vi "steuerprogramm-2.vi"() -> ()   [LabVIEW 2010]
uses:
  GVtdms.vi
  GVAbschalten.vi
  <vilib>/rvi/interface/nirviReadWriteControl/nirviReadWriteControl.xnode
  C:/Users/HAGAR-IV/Desktop/Zeugs/Johnny/pertrasgc fpga/fpga-programm-2.vi
  <vilib>/rvi/interface/nirviCloseFPGA/nirviCloseFPGA.xnode
  <vilib>/RVI Host/nirviSupport.llb/nirviErrorClusterFromErrorCode.vi
  <vilib>/rvi/errors/niLvFpgaWhatHappensToTopLevelVI.ctl
  <vilib>/rvi/interface/common/niFpgaNodeNameForErrorReporting.ctl
  <vilib>/rvi/errors/niLvFpgaAdjustHostInterfaceError.vi
  <vilib>/FPGAPlugInAG/cRIO-9114/niLvFpga_Close_cRIO-9114.vi
panel:
  in  "Pfad":path
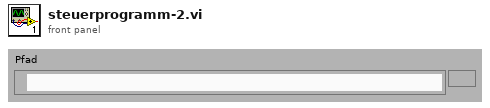
[diagram p1: front panel]
types:
  T1 = enum16{"open", "open or create", "create or replace", "create", "open (read-only)"}
  T2 = typedef "niFpgaNodeNameForErrorReporting.ctl" = enum16{"Open FPGA VI Reference", "Read/Write Control", "Invoke Method: Abort", "Invoke Method: Acknowledge IRQ", "Invoke Method: Download", "Invoke Method: FIFO.Configure", "Invoke Method: FIFO.Read", "Invoke Method: FIFO.Start", "Invoke Method: FIFO.Stop", "Invoke Method: FIFO.Write", "Invoke Method: Reset", "Invoke Method: Run", "Invoke Method: Wait on IRQ", "Close FPGA VI Reference"}
  T3 = typedef "niLvFpgaWhatHappensToTopLevelVI.ctl" = enum16{"top level VI scripted behind XNode", "top level VI inlined behind XNode"}
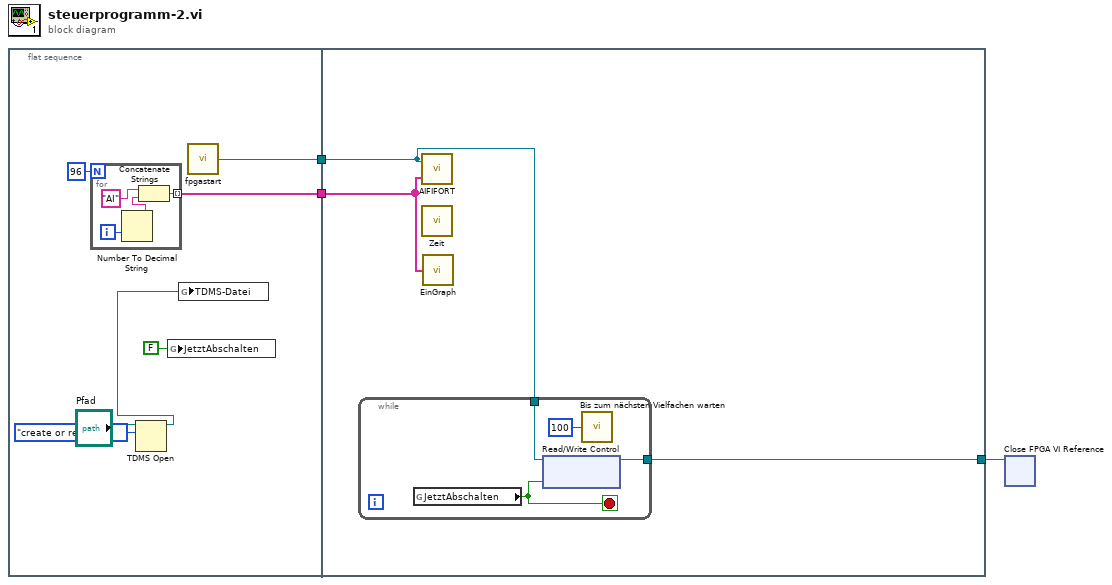
[diagram p0: block diagram]
diagram:
  n1 = flat-sequence {
    tunnel: [w10] -> w3
    tunnel: [w7] -> w1
    tunnel: w3 -> [w17]
    tunnel: [w16] -> w2
    tunnel: w1 -> [w15]
    frame #0 {
      n2 = for {
        N: 96 -> [_]
        tunnel: [w11] -> w7 mode=indexing
        i -> [w14]
        n3 = Number To Decimal String(number=w14) -> (decimal integer string=w12:string)  [unwired: 1 in]
        n4 = Concatenate Strings("AI", w12) -> (w11:string)
      }
      n5 = TDMS Open(10:T1."create or replace" ("Operation (0:Öffnen)"), 11:"Pfad") -> (3:w4:refnum<k34>)  [unwired: 4 in, 1 out]
      n6 = global write "GVAbschalten.vi" "JetztAbschalten"(FALSE ("JetztAbschalten")) -> ()
      n7 = global write "GVtdms.vi" "TDMS-Datei"(w4) -> ()
      n8 = call "fpgastart.vi"() -> ("FPGA VI Reference Out"=w10:refnum<k20>)  [unwired: 1 in]
    }
    frame #1 {
      n9 = while {
        tunnel: w17 -> [w21]
        tunnel: [w18] -> w16
        stop <- w20 stop-if-true
        n10 = global read "GVAbschalten.vi" "JetztAbschalten"() -> (w20:bool)
        n11 = xnode "Read/Write Control"("FPGA VI Reference In"=w21, "global stop"=w20) -> ("FPGA VI Reference Out"=w18:refnum<k20>)  [unwired: 1 in, 1 out]
        n12 = call "Bis zum nächsten Vielfachen warten"("Count(mSec)"=u32 100) -> ()  [unwired: 1 out]
      }
      n13 = call "AIFIFORT.vi"("AIsNamen"=w15, "FPGA VI Reference In"=w17) -> ()  [unwired: 1 in]
      n14 = call "Zeit.vi"() -> ()  [unwired: 12 in]
      n15 = call "EinGraph.vi"("AIs"=w15) -> ()  [unwired: 1 in]
    }
  }
  n16 = xnode "Close FPGA VI Reference"("FPGA VI Reference In"=w2) -> ()  [unwired: 1 in, 1 out]
